vi "Delete File.vi"(5 "Username":string, 6 "Password":string, 7 "Address":string, 8 "Error In":errorcluster) -> (0 "Error Out":errorcluster)   [LabVIEW 2018, in "Tests.lvlib" / "SFTP.lvlib"]
uses:
  SFTP.lvlib
  src/Toolkit/API/SFTP File/API/Typedefs/Flags.ctl
  <vilib>/addons/_JKI Toolkits/Caraya/classes/Test/Test.lvclass
  <vilib>/addons/_JKI Toolkits/Caraya/classes/Assert/Assert.lvclass
  src/Toolkit/API/SFTP/SFTP.lvclass
  src/Toolkit/API/SFTP File/SFTP File.lvclass
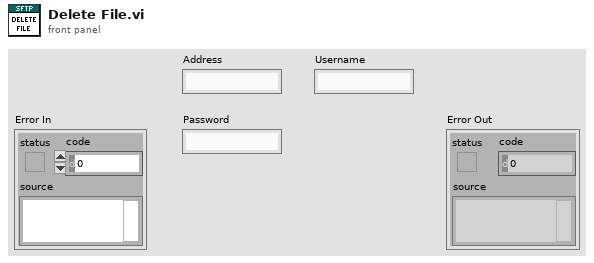
[diagram p1: front panel]
types:
  T1 = typedef "Toolkit.lvlib/SFTP File.lvclass/Flags.ctl" = cluster{"Read":bool, "Write":bool, "Append":bool, "Create":bool, "Truncate":bool, "Exclude":bool}
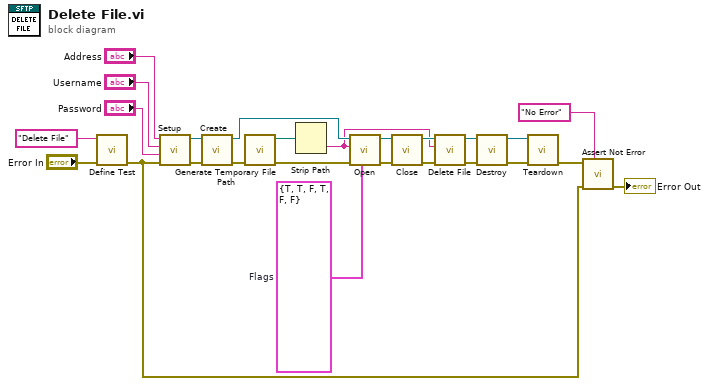
[diagram p0: block diagram]
diagram:
  w10 = T1 {"Read"=TRUE, "Write"=TRUE, "Append"=FALSE, "Create"=TRUE, "Truncate"=FALSE, "Exclude"=FALSE}  # Flags
  n1 = call <vilib>:"Define Test.vi"("error in (no error)"="Error In", "Label (VI Title)"="Delete File") -> ("error out"=w20:errorcluster)  [unwired: 9 in]
  n2 = call "Setup.vi"("Error In"=w20, "Password"="Password", "Username"="Username", "Address"="Address") -> ("Error Out"=w21:errorcluster, "Sesssion"=w16:refnum<class "Session.lvclass">)  [unwired: 6 in]
  n3 = call "Create.vi"("Error In"=w21, "Session"=w16) -> ("Error Out"=w9:errorcluster, "SFTP"=w8:refnum<class "SFTP.lvclass">)  [unwired: 8 in]
  n4 = call <vilib>:"Generate Temporary File Path.vi"("error in (no error)"=w9) -> ("error out"=w12:errorcluster, "Unique Temporary File Path"=w11:path)  [unwired: 9 in]
  n5 = Strip Path(path=w11) -> (name=w1:string)  [unwired: 1 out]
  n6 = call "Open.vi"("Flags"=w10, "Error In"=w12, "Remote Path"=w1, "SFTP"=w8) -> ("Error Out"=w6:errorcluster, "SFTP File"=w7:refnum<class "SFTP File.lvclass">)  [unwired: 6 in]
  n7 = call "Close.vi"("Error In"=w6, "SFTP File"=w7) -> ("Error Out"=w4:errorcluster, "SFTP"=w5:refnum<class "SFTP.lvclass">)  [unwired: 8 in]
  n8 = call "Delete File.vi"("Error In"=w4, "Remote Path"=w1, "SFTP In"=w5) -> ("Error Out"=w3:errorcluster, "SFTP Out"=w2:refnum<class "SFTP.lvclass">)  [unwired: 7 in]
  n9 = call "Destroy.vi"("Error In"=w3, "SFTP"=w2) -> ("Error Out"=w15:errorcluster, "Session"=w13:refnum<class "Session.lvclass">)  [unwired: 8 in]
  n10 = call "Teardown.vi"("Error In"=w15, "Session"=w13) -> ("Error Out"=w14:errorcluster)  [unwired: 9 in]
  n11 = call <vilib>:"Assert Not Error.vi"("Label"="No Error", "error in (no error)"=w20, "Not Error?"=w14) -> ("error out"=→"Error Out":errorcluster)  [unwired: 8 in]
